vi "GetROWSCOLON.vi"(11 "数组":string[](array[string])) -> (1 "布尔":bool, 2 "数值":dbl, 3 "数值 2":dbl)   [LabVIEW 2018]
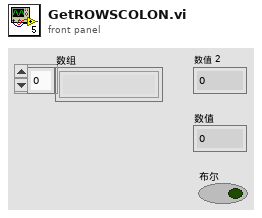
[diagram p1: front panel]
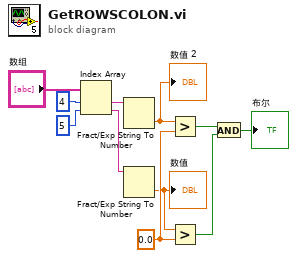
[diagram p0: block diagram]
diagram:
  w8 = 0.0
  n1 = Index Array(array="数组", index #1=4 ("索引"), index #2=5 ("索引")) -> (element #1=w4:string, element #2=w5:string)
  n2 = Fract/Exp String To Number(string=w4) -> (number=w6:dbl)  [unwired: 3 in, 1 out]
  "数值 2" <- w6
  n3 = Fract/Exp String To Number(string=w5) -> (number=w7:dbl)  [unwired: 3 in, 1 out]
  "数值" <- w7
  n4 = Greater?(x=w6, y=w8) -> (0:w10:bool)
  n5 = Greater?(x=w7, y=w8) -> (0:w9:bool)
  n6 = And(x=w10, y=w9) -> (x .and. y?=→"布尔":bool)
